vi "_toml_example.vi"() -> ()   [LabVIEW 2017]
uses:
  b87011d9-6f61-4e8a-a239-e3f8ce84dcb3.vi
  toml_lock_acquire.vi
  toml_lock_release.vi
  <vilib>/Utility/error.llb/Clear Errors.vi
  toml_lock_obtain.vi
  api/toml_api_is_loaded.vi
  api/toml_api_load.vi
  api/toml_api_get.vi
  api/toml_api_set.vi
  api/toml_api_dump.vi
panel:
  out "toml":string
  in  "data":T1={"booleans"={"bool"=FALSE, "bool with space"=TRUE}, "numbers"={"int"=123, "int with space"=-123, "uint"=123, "uint with space"=27893, "dbl"=3.1415, "dbl with space"=-1.52e-05, "0x.uint as hex"=3735928559, "0b.uint as binary"=26, "0o.uint as octal"=4294967295}, "strings"={"string"="hello world", "multi line string"="line 1\nline 2", "'.literal string"="", "'''.multi line literal"="", "paths are always literals"=path "", "string escape charaters"="hello world"}, "datetime"={"date and time"=timestamp(3647394845.8848343 s since 1904-01-01), "0D.date only"=timestamp(2625418800 s since 1904-01-01), "0T.time only"=timestamp(3029624132.123 s since 1904-01-01)}} {"numbers"."0o.uint as octal" format="%0o"; "numbers"."0b.uint as binary" format="%032b"; "numbers"."0x.uint as hex" format="%08x"}
  out "error out":errorcluster
  out "exists_setdefault":bool
  # "Special label prefixes:\n0x.  = hex\n0b. = binary\n0o. = octal\n'. = literal string\n'''. = multi-line literal string\n0D. = date only\n0T. = time only"
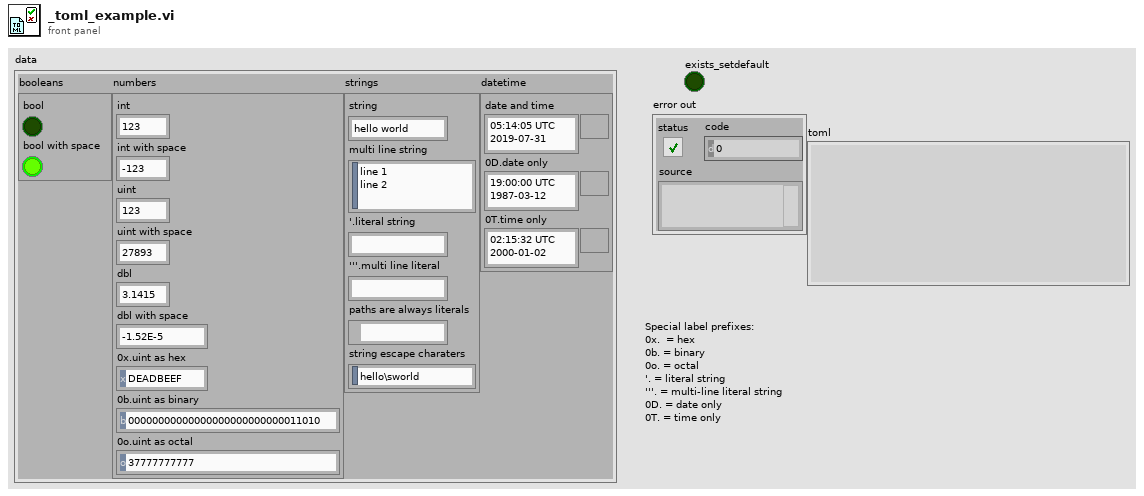
[diagram p1: front panel]
types:
  T1 = cluster{"booleans":cluster{"bool":bool, "bool with space":bool}, "numbers":cluster{"int":i32, "int with space":i32, "uint":u32, "uint with space":u32, "dbl":dbl, "dbl with space":dbl, "0x.uint as hex":u32, "0b.uint as binary":u32, "0o.uint as octal":u32}, "strings":cluster{"string":string, "multi line string":string, "'.literal string":string, "'''.multi line literal":string, "paths are always literals":path, "string escape charaters":string}, "datetime":cluster{"date and time":timestamp, "0D.date only":timestamp, "0T.time only":timestamp}}
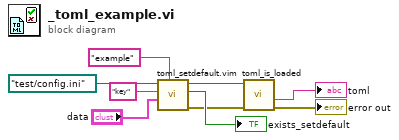
[diagram p0: block diagram]
diagram:
  n1 = call "toml_setdefault.vim"("section"="example", "default"="data", "key"="key", "path in"=path "test/config.ini") -> ("error out"=w5:errorcluster, "key exists"=→"exists_setdefault":bool, "path out"=w3:path)  [unwired: 4 in, 1 out]
  n2 = call "toml_is_loaded.vi"("error in (no error)"=w5, "path in"=w3) -> ("error out"=→"error out":errorcluster, "toml"=→"toml":string)  [unwired: 6 in, 2 out]
